vi "Test Queue Synch 2.vi"() -> ()   [LabVIEW 2021]
uses:
  Source/Support/Nodes/abs_Node/Status.ctl
  Source/System/bt_System.lvclass
  Source/Support/Nodes/Decorators/Repeater/Support/Finish On - Type.ctl
  Source/Support/Nodes/Composites/abs_Parallel/Support/Status Calculation.ctl
  Source/Blackboard/Blackboard.lvclass
  Source/Blackboard/Support/Filter Type.ctl
  Source/Blackboard/Blackboard.lvclass/Blackboard.ctl
  Source/Support/Nodes/Leaves/abs_Type Leaf/abs_Type Leaf.lvclass/abs_Type Leaf.ctl
  Source/Blackboard/Get Value Type/Get I32.vi
  <vilib>/TSA/Abstract Data Classes/Abs_Types/I32 Integer/Static Read.vi
  Source/Blackboard/Support/Index Group.vi
  Source/Blackboard/Support/Index Tags.vi
  Source/Support/Nodes/Leaves/abs_Type Leaf/Properties/Write Value Class.vi
  <vilib>/TSA/Omni-Bus/Local Bus/Support/I32/Local Bus_I32.lvclass
  C:/Program Files (x86)/National Instruments/LabVIEW 2021/vi.lib/TSA/Abstract Data Classes/Abs_Types/Value/Abs_Value.lvclass
  <vilib>/TSA/Abstract Data Classes/Abs_Types/I32 Integer/Abs_I32 Integer.lvclass
  C:/Program Files (x86)/National Instruments/LabVIEW 2021/vi.lib/TSA/Abstract Data Classes/Abs_Types/Numeric/Abs_Numeric.lvclass
  Source/Support/Nodes/Leaves/Synch/Queue/Send/bt_Send_Queue.lvclass
  C:/Users/Tim/Documents/GitHub/LV_Behaviour_Tree/Source/Support/Nodes/abs_Node/bt_Node.lvclass
  Source/Support/Nodes/Leaves/Test Boolean/Test Abs_Boolean.lvclass
  C:/Users/Tim/Documents/GitHub/LV_Behaviour_Tree/Source/Support/Nodes/Leaves/abs_Type Leaf/abs_Type Leaf.lvclass
  <vilib>/TSA/Abstract Data Classes/Abs_Types/Boolean/Abs_Boolean.lvclass
  C:/Program Files (x86)/National Instruments/LabVIEW 2021/vi.lib/TSA/Abstract Data Classes/Abs_Types/Type/Abs_Type.lvclass
  Source/Support/Nodes/Leaves/Synch/Queue/WaitOn/bt_WaitOn_Queue.lvclass
  <vilib>/TSA/Omni-Bus/Local Bus/Support/Initialise DVR's.vi
  <vilib>/TSA/Abstract Data Classes/Functions/Math/Support/Increment/I32/Method.vi
  <vilib>/TSA/Abstract Data Classes/Constants/Support/I32/I32.vi
  <vilib>/TSA/Abstract Data Classes/Functions/Compare/Support/Greater Equal/I32/Method.vi
  <vilib>/TSA/Abstract Data Classes/Abs_Types/Value/Abs_Value.lvclass
  <vilib>/TSA/Abstract Data Classes/Abs_Types/Type/Abs_Type.lvclass
  <vilib>/TSA/Omni-Bus/Local Bus/Support/DBL/Local Bus_DBL.lvclass
  <vilib>/TSA/Omni-Bus/Local Bus/Support/SGL/Local Bus_SGL.lvclass
  <vilib>/TSA/Omni-Bus/Local Bus/Support/EXT/Local Bus_EXT.lvclass
  <vilib>/TSA/Omni-Bus/Local Bus/Support/Bool/Local Bus_Boolean.lvclass
  <vilib>/TSA/Omni-Bus/Local Bus/Support/STR/Local Bus_String.lvclass
  <vilib>/TSA/Omni-Bus/Local Bus/Support/Variant/Local Bus_Variant.lvclass
  <vilib>/TSA/Omni-Bus/Local Bus/Support/WFM/Local Bus_Waveform.lvclass
  <vilib>/TSA/Omni-Bus/Local Bus/Support/Time/Local Bus_Time.lvclass
  <vilib>/TSA/Omni-Bus/Local Bus/Support/U8/Local Bus_U8.lvclass
  <vilib>/TSA/Omni-Bus/Local Bus/Support/U16/Local Bus_U16.lvclass
  <vilib>/TSA/Omni-Bus/Local Bus/Support/U32/Local Bus_U32.lvclass
  <vilib>/TSA/Omni-Bus/Local Bus/Support/U64/Local Bus_U64.lvclass
  <vilib>/TSA/Omni-Bus/Local Bus/Support/I8/Local Bus_I8.lvclass
  <vilib>/TSA/Omni-Bus/Local Bus/Support/I16/Local Bus_I16.lvclass
  <vilib>/TSA/Omni-Bus/Local Bus/Support/I64/Local Bus_I64.lvclass
  <vilib>/TSA/Omni-Bus/Local Bus/Support/CSGL/Local Bus_CSGL.lvclass
  <vilib>/TSA/Omni-Bus/Local Bus/Support/CDBL/Local Bus_CDBL.lvclass
  <vilib>/TSA/Omni-Bus/Local Bus/Support/CEXT/Local Bus_CEXT.lvclass
  <vilib>/TSA/Omni-Bus/Local Bus/Support/Type/Local Bus_Type.lvclass
  Source/BT.lvlib
  Source/Support/Nodes/Composites/abs_Parallel/bt_Parallel.lvclass
  Source/Support/Nodes/Decorators/Repeater/bt_Repeater.lvclass
  C:/Program Files (x86)/National Instruments/LabVIEW 2021/vi.lib/TSA/Abstract Data Classes/Abs_Types/Integer/Abs_Integer.lvclass
  C:/Program Files (x86)/National Instruments/LabVIEW 2021/vi.lib/TSA/Abstract Data Classes/Abs_Types/I32 Integer/Abs_I32 Integer.lvclass
  <vilib>/TSA/Abstract Data Classes/Functions/Math/Support/Increment/I32/Increment_I32.lvclass
  <vilib>/TSA/Abstract Data Classes/Constants/Support/I32/Const_I32.lvclass
  <vilib>/TSA/Abstract Data Classes/Functions/Compare/Support/Greater Equal/I32/Greater Equal_I32.lvclass
  C:/Users/Tim/Documents/GitHub/LV_Behaviour_Tree/Source/Support/Nodes/Leaves/Synch/With Values/Send/bt_Send_Synch_WithValues.lvclass
  C:/Users/Tim/Documents/GitHub/LV_Behaviour_Tree/Source/Support/Nodes/Leaves/Synch/Parent/Send/bt_Send_Synch.lvclass
  C:/Users/Tim/Documents/GitHub/LV_Behaviour_Tree/Source/Support/Nodes/Leaves/Leaf/bt_Leaf.lvclass
  C:/Users/Tim/Documents/GitHub/LV_Behaviour_Tree/Source/Support/Nodes/Leaves/Synch/Queue/Send/bt_Send_Queue.lvclass
  C:/Users/Tim/Documents/GitHub/LV_Behaviour_Tree/Source/Support/Nodes/Leaves/Synch/With Values/WaitOn/bt_WaitOn_Synch_WithValues.lvclass
  C:/Users/Tim/Documents/GitHub/LV_Behaviour_Tree/Source/Support/Nodes/Leaves/Synch/Parent/WaitOn/bt_WaitOn_Synch.lvclass
  C:/Users/Tim/Documents/GitHub/LV_Behaviour_Tree/Source/Support/Nodes/Leaves/Synch/Queue/WaitOn/bt_WaitOn_Queue.lvclass
  Source/Support/Nodes/abs_Node/bt_Node.lvclass
panel:
  out "Groups":string[](array[string])
  out "Fail Count":u32
  out "Tags":string[](array[string])
  out "Success Count":u32
  out "i":u32
  out "n":u32
  out "error out 5":errorcluster
  in  "stop":bool
  out "Status":T1
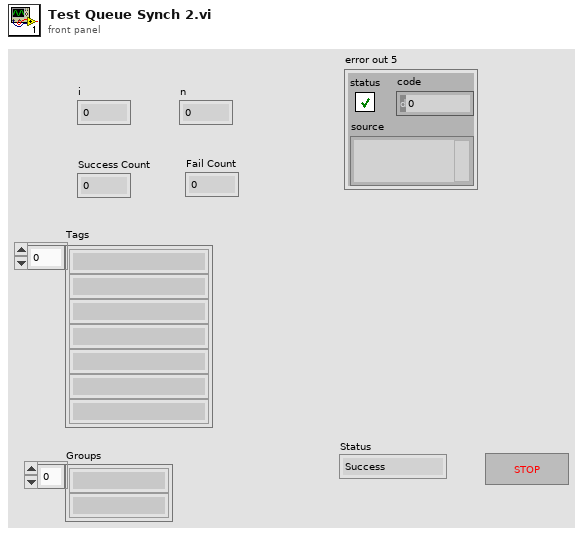
[diagram p1: front panel]
types:
  T1 = typedef "BT.lvlib/bt_Node.lvclass/Status.ctl" = enum16{"Success", "Failure", "Running"}
  T2 = typedef "BT.lvlib/bt_Repeater.lvclass/Finish On - Type.ctl" = enum16{"Success", "Failure", "Never"}
  T3 = typedef "Blackboard.lvclass/Filter Type.ctl" = enum16{"All Tags", "NI Specific Type", "Boolean", "String", "Numeric", "Float", "Integer"}
  T4 = typedef "BT.lvlib/bt_Parallel.lvclass/Status Calculation.ctl" = enum16{"Succeed on All Succeed", "Failure on All Failure", "Succeed on Any Succeed", "Failure on Any Failure"}
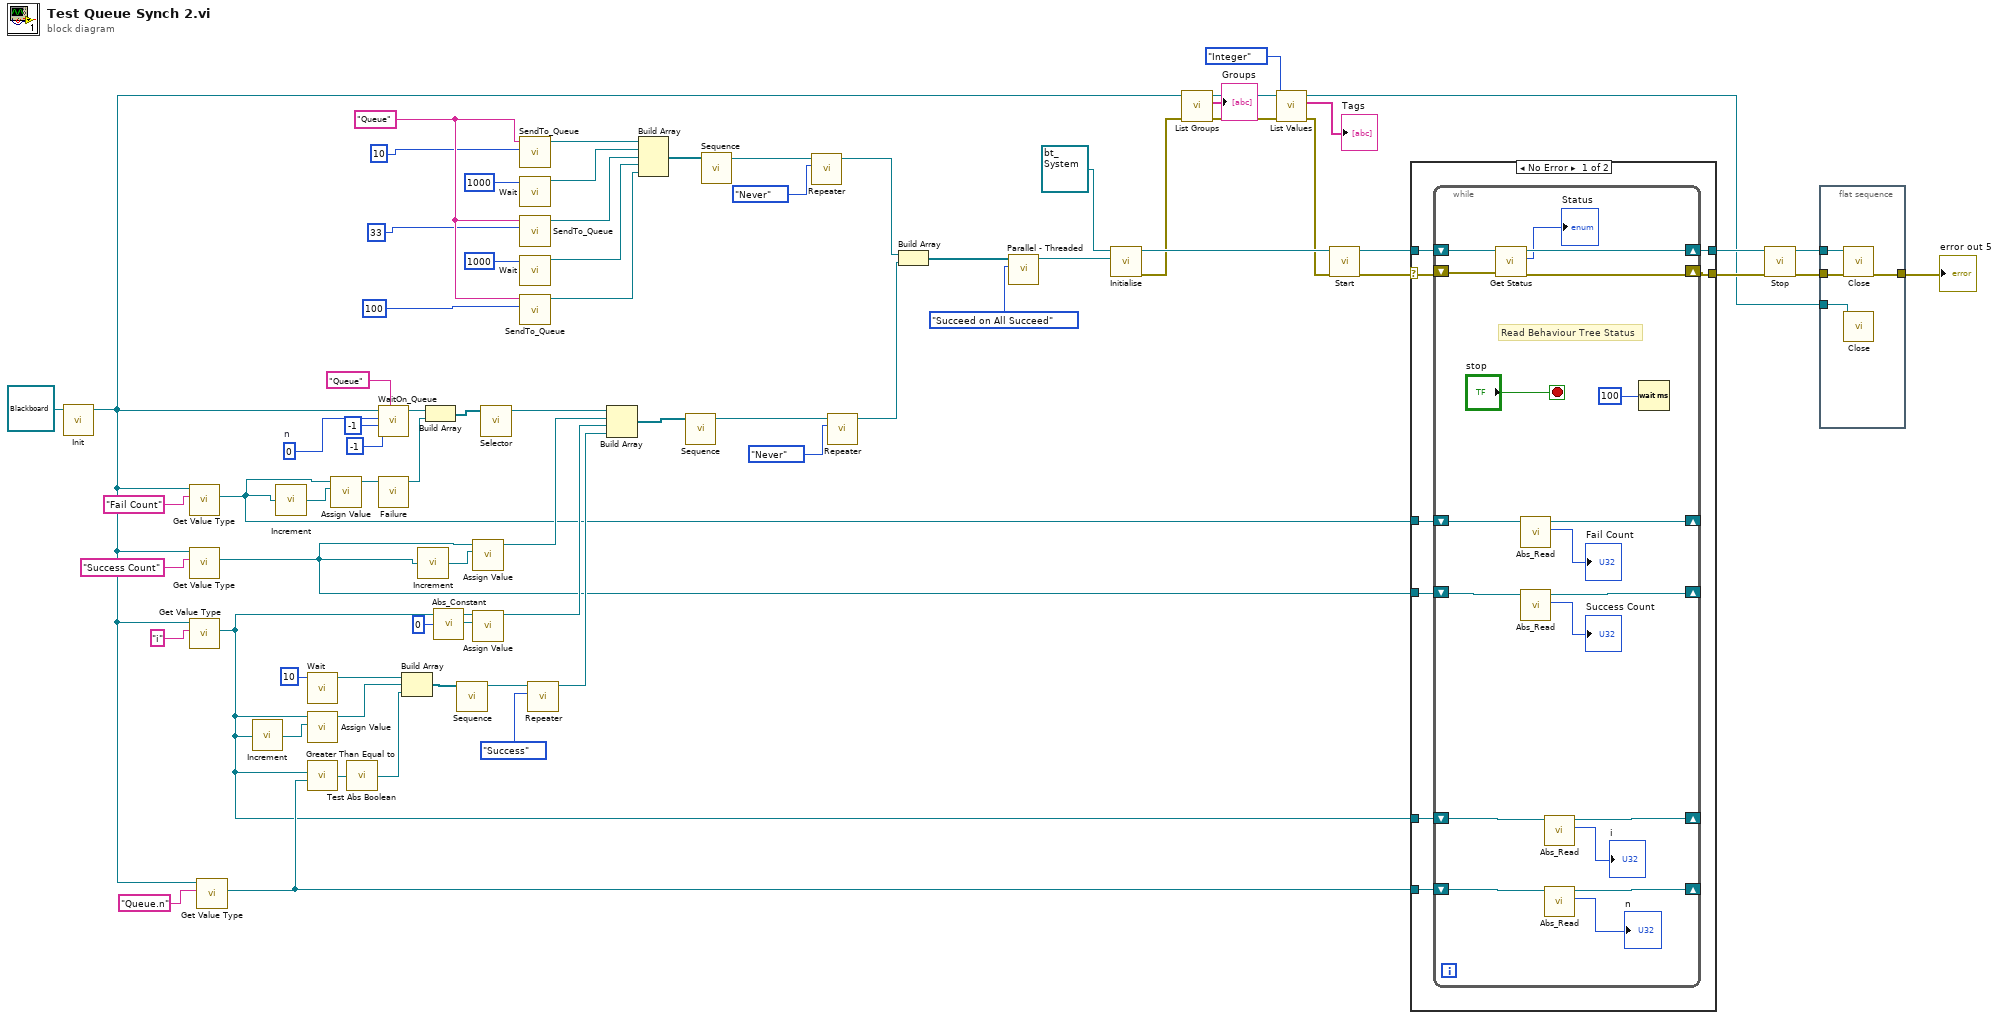
[diagram p0: block diagram]
diagram:
  w46 = 0  # n
  w53 = "Queue" ("Name")
  n1 = call-dynamic "Init.vi"("bt_Blackboard in"=refnum<class "Blackboard.lvclass"> refnum) -> ("bt_Blackboard out"=w9:refnum<class "Blackboard.lvclass">)  [unwired: 9 in, 1 out]
  n2 = call-poly "Get Value Type.vi"("Tag"="Fail Count", "Blackboard in"=w9) -> ("Value"=w10:refnum<class "Abs_I32 Integer.lvclass">)  [unwired: 6 in, 3 out]
  n3 = call-poly "Get Value Type.vi"("Tag"="Success Count", "Blackboard in"=w9) -> ("Value"=w23:refnum<class "Abs_I32 Integer.lvclass">)  [unwired: 6 in, 3 out]
  n4 = call-poly "Get Value Type.vi"("Tag"="i", "Blackboard in"=w9) -> ("Value"=w30:refnum<class "Abs_I32 Integer.lvclass">)  [unwired: 6 in, 3 out]
  n5 = call-poly "Get Value Type.vi"("Tag"="Queue.n", "Blackboard in"=w9) -> ("Value"=w32:refnum<class "Abs_I32 Integer.lvclass">)  [unwired: 6 in, 3 out]
  n6 = call-poly <vilib>:"Increment.vi"("Value"=w30) -> ("Result"=w36:refnum<class "Abs_I32 Integer.lvclass">)  [unwired: 4 in]
  n7 = call-poly <vilib>:"Increment.vi"("Value"=w10) -> ("Result"=w15:refnum<class "Abs_I32 Integer.lvclass">)  [unwired: 4 in]
  n8 = call "Wait.vi"("Time (ms)"=u32 10) -> ("Node Out"=w29:refnum<class "bt_Node.lvclass">)  [unwired: 10 in]
  n9 = call "Assign Value.vi"("Assigned Value"=w36, "Value"=w30) -> ("Node Out"=w35:refnum<class "bt_Node.lvclass">)  [unwired: 9 in]
  n10 = call-poly <vilib>:"Greater Than Equal to.vi"("Value B"=w32, "Value A"=w30) -> ("Result"=w34:refnum<class "Abs_Boolean.lvclass">)  [unwired: 4 in]
  n11 = call "Assign Value.vi"("Assigned Value"=w15, "Value"=w10) -> ("Node Out"=w12:refnum<class "bt_Node.lvclass">)  [unwired: 9 in]
  n12 = call "Test Abs Boolean.vi"("Abs_Boolean.lvclass"=w34) -> ("abs_Node"=w33:refnum<class "bt_Node.lvclass">)  [unwired: 4 in]
  n13 = call "WaitOn_Queue.vi"("Queue Name"="Queue" ("Name"), "Max Queue Size"=-1, "Timeout (ms)"=-1, "Message Type"=w46, "bt_Blackboard in"=w9) -> ("Queue out"=w14:refnum<class "bt_WaitOn_Queue.lvclass">)  [unwired: 5 in, 1 out]
  n14 = call "Failure.vi"("Node In"=w12) -> ("Node"=w11:refnum<class "bt_Node.lvclass">)  [unwired: 10 in]
  n15 = Build Array(w29, w35, w33) -> (w41:refnum<class "bt_Node.lvclass">[])
  n16 = call-poly <vilib>:"Increment.vi"("Value"=w23) -> ("Result"=w26:refnum<class "Abs_I32 Integer.lvclass">)  [unwired: 4 in]
  n17 = Build Array(w14, w11) -> (w13:refnum<class "bt_Node.lvclass">[])
  n18 = call-poly <vilib>:"Abs_Constant.vi"("Value"=0 ("n")) -> ("Constant"=w37:refnum<class "Abs_I32 Integer.lvclass">)  [unwired: 4 in]
  n19 = call "Sequence.vi"("Nodes"=w41) -> ("Node"=w42:refnum<class "bt_Node.lvclass">)  [unwired: 10 in]
  n20 = call "Assign Value.vi"("Assigned Value"=w26, "Value"=w23) -> ("Node Out"=w25:refnum<class "bt_Node.lvclass">)  [unwired: 9 in]
  n21 = call "Assign Value.vi"("Assigned Value"=w37, "Value"=w30) -> ("Node Out"=w31:refnum<class "bt_Node.lvclass">)  [unwired: 9 in]
  n22 = call "Selector.vi"("Nodes"=w13) -> ("Node"=w17:refnum<class "bt_Node.lvclass">)  [unwired: 10 in]
  n23 = call "SendTo_Queue.vi"("Message"=10, "Queue Name"=w53) -> ("Queue Out"=w65:refnum<class "bt_Send_Queue.lvclass">)  [unwired: 9 in]
  n24 = call "Wait.vi"("Time (ms)"=u32 1000) -> ("Node Out"=w60:refnum<class "bt_Node.lvclass">)  [unwired: 10 in]
  n25 = call "SendTo_Queue.vi"("Message"=33, "Queue Name"=w53) -> ("Queue Out"=w63:refnum<class "bt_Send_Queue.lvclass">)  [unwired: 9 in]
  n26 = call "Wait.vi"("Time (ms)"=u32 1000) -> ("Node Out"=w58:refnum<class "bt_Node.lvclass">)  [unwired: 10 in]
  n27 = call "SendTo_Queue.vi"("Message"=100, "Queue Name"=w53) -> ("Queue Out"=w62:refnum<class "bt_Send_Queue.lvclass">)  [unwired: 9 in]
  n28 = call "Repeater.vi"("Finish On"=Finish_On_-_Type."Success", "Node In"=w42) -> ("Node Out"=w43:refnum<class "bt_Node.lvclass">)  [unwired: 9 in]
  n29 = Build Array(w17, w25, w31, w43) -> (w45:refnum<class "bt_Node.lvclass">[])
  n30 = Build Array(w65, w60, w63, w58, w62) -> (w64:refnum<class "bt_Node.lvclass">[])
  n31 = call "Sequence.vi"("Nodes"=w45) -> ("Node"=w44:refnum<class "bt_Node.lvclass">)  [unwired: 10 in]
  n32 = call "Sequence.vi"("Nodes"=w64) -> ("Node"=w2:refnum<class "bt_Node.lvclass">)  [unwired: 10 in]
  n33 = call "Repeater.vi"("Finish On"=Finish_On_-_Type."Never", "Node In"=w2) -> ("Node Out"=w1:refnum<class "bt_Node.lvclass">)  [unwired: 9 in]
  n34 = call "Repeater.vi"("Finish On"=Finish_On_-_Type."Never", "Node In"=w44) -> ("Node Out"=w56:refnum<class "bt_Node.lvclass">)  [unwired: 9 in]
  n35 = Build Array(w1, w56) -> (w67:refnum<class "bt_Node.lvclass">[])
  n36 = call "Parallel - Threaded.vi"("Status Calculation"=Status_Calculation."Succeed on All Succeed", "Nodes"=w67) -> ("Node"=w66:refnum<class "bt_Node.lvclass">)  [unwired: 9 in]
  n37 = call "Initialise.vi"("Behaviour Tree"=w66, "bt_System in"=refnum<class "bt_System.lvclass"> refnum) -> ("error out"=w7:errorcluster, "bt_System out"=w21:refnum<class "bt_System.lvclass">)  [unwired: 8 in]
  n38 = call "List Groups.vi"("error in (no error)"=w7, "Blackboard in"=w9) -> ("error out"=w6:errorcluster, "Groups"=→"Groups":string[], "Blackboard out"=w8:refnum<class "Blackboard.lvclass">)  [unwired: 7 in]
  n39 = call "List Values.vi"("error in (no error)"=w6, "Broad Types"=Filter_Type."Integer", "Blackboard in"=w8) -> ("error out"=w20:errorcluster, "Tags"=→"Tags":string[], "Blackboard out"=w19:refnum<class "Blackboard.lvclass">)  [unwired: 5 in, 1 out]
  n40 = call "Start.vi"("error in (no error)"=w20, "bt_System in"=w21) -> ("error out"=w52:errorcluster, "bt_System out"=w73:refnum<class "bt_System.lvclass">)  [unwired: 8 in]
  n41 = case shown="No Error" w52 {
    selector: w52 -> [w79 w102]
    tunnel: w73 -> [w82 w103]
    tunnel: [w81 w103] -> w70
    tunnel: w32 -> [w80 _]
    tunnel: [w78 w102] -> w50
    tunnel: w30 -> [w77 _]
    tunnel: w23 -> [w76 _]
    tunnel: w10 -> [w75 _]
    frame No Error {
      n42 = while {
        shift-right: [w99] -> w81
        shift-left: w82 -> [w100]
        shift-right: [w93] -> _
        shift-left: w80 -> [w94]
        shift-right: [w95] -> w78
        shift-left: w79 -> [w96]
        shift-right: [w90] -> _
        shift-left: w77 -> [w89]
        shift-right: [w87] -> _
        shift-left: w76 -> [w88]
        shift-right: [w84] -> _
        shift-left: w75 -> [w83]
        stop <- "stop" stop-if-true
        # "Read Behaviour Tree Status"
        n43 = call "Get Status.vi"("error in (no error)"=w96, "bt_System in"=w100) -> ("error out"=w95:errorcluster, "Status"=→"Status":T1, "bt_System out"=w99:refnum<class "bt_System.lvclass">)  [unwired: 7 in]
        n44 = call-poly <vilib>:"Abs_Read.vi"("Abs_I32 Integer in"=w83) -> ("Value"=→"Fail Count":i32, "Abs_I32 Integer out"=w84:refnum<class "Abs_I32 Integer.lvclass">)  [unwired: 8 in, 1 out]
        n45 = call-poly <vilib>:"Abs_Read.vi"("Abs_I32 Integer in"=w88) -> ("Value"=→"Success Count":i32, "Abs_I32 Integer out"=w87:refnum<class "Abs_I32 Integer.lvclass">)  [unwired: 8 in, 1 out]
        n46 = call-poly <vilib>:"Abs_Read.vi"("Abs_I32 Integer in"=w89) -> ("Value"=→"i":i32, "Abs_I32 Integer out"=w90:refnum<class "Abs_I32 Integer.lvclass">)  [unwired: 8 in, 1 out]
        n47 = call-poly <vilib>:"Abs_Read.vi"("Abs_I32 Integer in"=w94) -> ("Value"=→"n":i32, "Abs_I32 Integer out"=w93:refnum<class "Abs_I32 Integer.lvclass">)  [unwired: 8 in, 1 out]
        n48 = Wait (ms)(milliseconds to wait=u32 100) -> ()  [unwired: 1 out]
      }
    }
    frame Error {
    }
  }
  n49 = call "Stop.vi"("error in (no error)"=w50, "bt_System in"=w70) -> ("error out"=w71:errorcluster, "bt_System out"=w72:refnum<class "bt_System.lvclass">)  [unwired: 8 in]
  n50 = flat-sequence {
    tunnel: w72 -> [w107]
    tunnel: w71 -> [w106]
    tunnel: [w105] -> w51
    tunnel: w19 -> [w104]
    frame #0 {
      n51 = call-dynamic "Close.vi"("error in (no error)"=w106, "bt_System in"=w107) -> ("error out"=w105:errorcluster)  [unwired: 8 in, 1 out]
      n52 = call-dynamic "Close.vi"("bt_Blackboard in"=w104) -> ()  [unwired: 9 in, 2 out]
    }
  }
  "error out 5" <- w51
